vi "绘制方块(多块).vi"(8 "偏移量 2":cluster{"X":i32, "Y":i32}, 9 "偏移量":cluster{"X":i32, "Y":i32}, 10 "数组 2":u32[][](array[colorbox]), 11 "数组":u32[][](array[colorbox])) -> (3 "数组 3":u32[][](array[colorbox]))   [LabVIEW 2012]
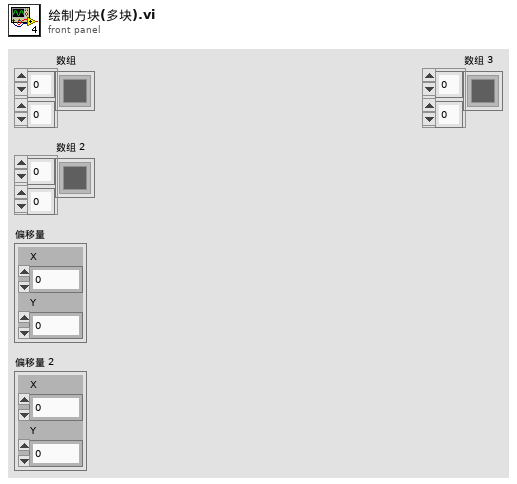
[diagram p1: front panel]
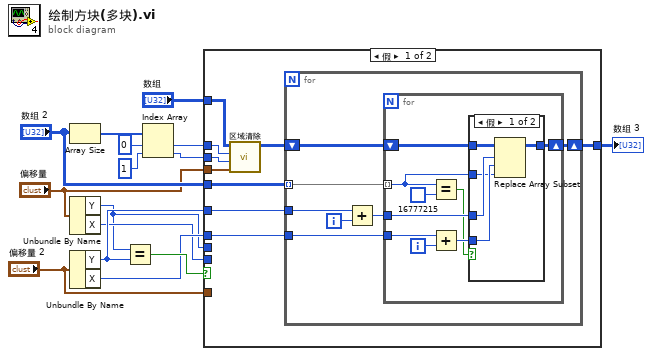
[diagram p0: block diagram]
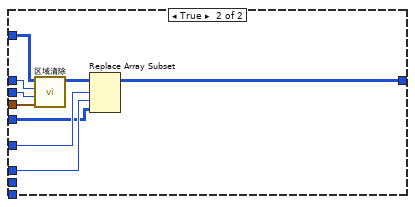
[diagram p3: hidden frame]
diagram:
  n1 = Array Size(array="数组 2") -> (size(s)=w15:i32[])
  n2 = Unbundle By Name("偏移量") -> ("Y"=w4:i32, "X"=w5:i32)
  n3 = Unbundle By Name("偏移量 2") -> ("Y"=w6:i32, "X"=w7:i32)
  n4 = Equal?(x=w4, y=w6) -> (x = y?=w12:bool)
  n5 = Index Array(array=w15, index #1=0 ("索引"), index #2=1 ("索引")) -> (element #1=w8:i32, element #2=w9:i32)
  n6 = case shown="假" w12 {
    tunnel: "数组" -> [w24 w55]
    tunnel: "数组 2" -> [w20 w48]
    tunnel: w9 -> [w22 w53]
    tunnel: w8 -> [w23 w54]
    tunnel: w7 -> [w18 w49]
    tunnel: w6 -> [w19 w50]
    tunnel: w5 -> [_ _]
    tunnel: w4 -> [_ _]
    tunnel: "偏移量" -> [w21 w52]
    tunnel: "偏移量 2" -> [_ _]
    tunnel: [w16 w47] -> w1
    frame False {
      n7 = call "区域清除.vi"("偏移量"=w21, "列"=w22, "行"=w23, "数组"=w24) -> ("数组 3"=w17:u32[][])  [unwired: 7 in]
      n8 = for {
        tunnel: w20 -> [w31] mode=indexing
        tunnel: w19 -> [w28]
        tunnel: w18 -> [w30]
        shift-right: [w25] -> w16
        shift-left: w17 -> [w29]
        i -> [w27]
        n9 = Add(x=w28, y=w27) -> (x+y=w26:i32)
        n10 = for {
          tunnel: w31 -> [w33] mode=indexing
          tunnel: w30 -> [w39]
          tunnel: w26 -> [w40]
          shift-right: [w32] -> w25
          shift-left: w29 -> [w36]
          i -> [w38]
          n11 = Equal?(x=w33, y=u32 16777215) -> (x = y?=w34:bool)
          n12 = Add(x=w39, y=w38) -> (x+y=w37:i32)
          n13 = case shown="假" w34 {
            tunnel: w36 -> [w45 w46]
            tunnel: w40 -> [w44 _]
            tunnel: w37 -> [w43 _]
            tunnel: w33 -> [w42 _]
            tunnel: [w41 w46] -> w32
            frame False {
              n14 = Replace Array Subset(array=w45, new element=w42, index (row)=w44, index (col)=w43) -> (w41:u32[][])
            }
            frame True {
            }
          }
        }
      }
    }
    frame True {
      n15 = call "区域清除.vi"("偏移量"=w52, "列"=w53, "行"=w54, "数组"=w55) -> ("数组 3"=w51:u32[][])  [unwired: 7 in]
      n16 = Replace Array Subset(array=w51, new element=w48, index (row)=w50, index (col)=w49) -> (w47:u32[][])
    }
  }
  "数组 3" <- w1
